vi "7HP_Create datalog header string.vi"() -> (0 "Datalog header string":string)   [LabVIEW 2021]
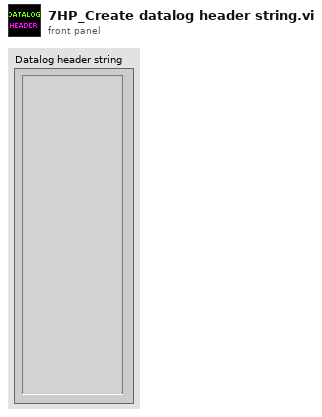
[diagram p1: front panel]
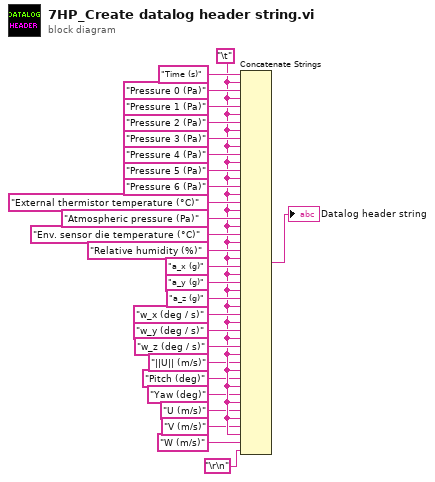
[diagram p0: block diagram]
diagram:
  w8 = "\t"
  n1 = Concatenate Strings("Time (s)", w8, "Pressure 0 (Pa)", w8, "Pressure 1 (Pa)", w8, "Pressure 2 (Pa)", w8, "Pressure 3 (Pa)", w8, "Pressure 4 (Pa)", w8, "Pressure 5 (Pa)", w8, "Pressure 6 (Pa)", w8, "External thermistor temperature (°C)", w8, "Atmospheric pressure (Pa)", w8, "Env. sensor die temperature (°C)", w8, "Relative humidity (%)", w8, "a_x (g)", w8, "a_y (g)", w8, "a_z (g)", w8, "w_x (deg / s)", w8, "w_y (deg / s)", w8, "w_z (deg / s)", w8, "||U|| (m/s)", w8, "Pitch (deg)", w8, "Yaw (deg)", w8, "U (m/s)", w8, "V (m/s)", w8, "W (m/s)", "\r\n") -> (→"Datalog header string":string)
